vi "FTW-Listener-Wait On Connection.vi"(0 "Gmsg_Listener In":refnum<class "FTW-Listener.lvclass">, 11 "error in":errorcluster) -> (4 "Gmsg_Listener Out":refnum<class "FTW-Listener.lvclass">, 6 "Endpoint":refnum<class "FTW-Endpoint.lvclass">, 15 "error out":errorcluster)   [LabVIEW 2013, in "FTW-Listener.lvclass"]
uses:
  FTW-Listener.lvclass
  Endpoint/FTW-Endpoint.lvclass
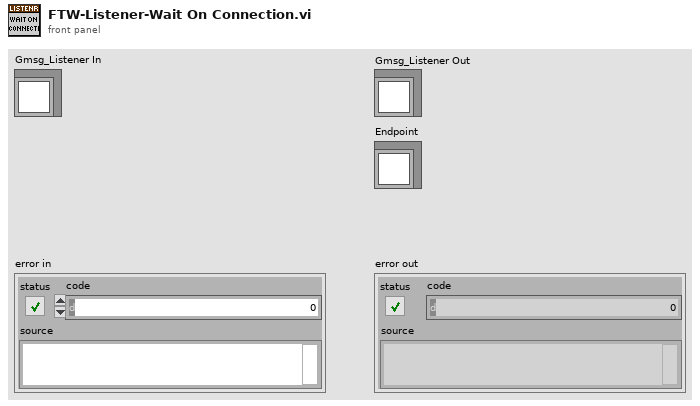
[diagram p1: front panel]
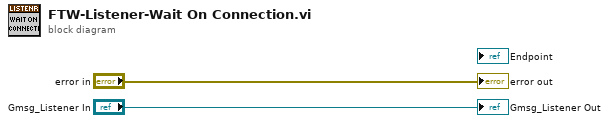
[diagram p0: block diagram]
diagram:
  "Gmsg_Listener Out" <- "Gmsg_Listener In"
  "error out" <- "error in"
